vi "Sensors.vi"() -> ()   [LabVIEW 2017]
uses:
  <vilib>/DAQmx/read.llb/DAQmx Read (Analog 1D Wfm NChan 1Samp).vi
  <vilib>/DAQmx/read.llb/DAQmx Read (Analog 1D Wfm NChan NSamp).vi
  <vilib>/DAQmx/miscellaneous.llb/DAQmx Fill In Error Info.vi
panel:
  out "output cluster":T1={"Dynamic Data"=[{"t0"=timestamp(0 s since 1904-01-01), "dt"=1.0, "Y"=[14.93], "attributes"=variant("Alicat_unit"=variant(string "PSIA"), "NI_ChannelName"=variant(string "Absolute Pressure_O2"), "NI_UnitDescription"=variant(string "psi"))}, {"t0"=timestamp(0 s since 1904-01-01), "dt"=1.0, "Y"=[18.45], "attributes"=variant("Alicat_unit"=variant(string "°C"), "NI_ChannelName"=variant(string "Temperature_O2"), "NI_UnitDescription"=variant(string "degC"))}, {"t0"=timestamp(0 s since 1904-01-01), "dt"=1.0, "Y"=[-0.1], "attributes"=variant("Alicat_unit"=variant(string "LPM"), "NI_ChannelName"=variant(string "Volumetric Flow_O2"), "NI_UnitDescription"=variant(string "l/min"))}, {"t0"=timestamp(0 s since 1904-01-01), "dt"=1.0, "Y"=[-0.1], "attributes"=variant("Alicat_unit"=variant(string "SLPM"), "NI_ChannelName"=variant(string "Mass Flow_O2"), "NI_UnitDescription"=variant(string "kg/min"))}, {"t0"=timestamp(0 s since 1904-01-01), "dt"=1.0, "Y"=[104.12], "attributes"=variant("Alicat_unit"=variant(string "PSIA"), "NI_ChannelName"=variant(string "Absolute Pressure_Ar"), "NI_UnitDescription"=variant(string "psi"))}, {"t0"=timestamp(0 s since 1904-01-01), "dt"=1.0, "Y"=[18.33], "attributes"=variant("Alicat_unit"=variant(string "°C"), "NI_ChannelName"=variant(string "Temperature_Ar"), "NI_UnitDescription"=variant(string "degC"))}, {"t0"=timestamp(0 s since 1904-01-01), "dt"=1.0, "Y"=[-0.01], "attributes"=variant("Alicat_unit"=variant(string "LPM"), "NI_ChannelName"=variant(string "Volumetric Flow_Ar"), "NI_UnitDescription"=variant(string "l/min"))}, {"t0"=timestamp(0 s since 1904-01-01), "dt"=1.0, "Y"=[-0.09], "attributes"=variant("Alicat_unit"=variant(string "SLPM"), "NI_ChannelName"=variant(string "Mass Flow_Ar"), "NI_UnitDescription"=variant(string "kg/min"))}, {"t0"=timestamp(3595264812.029535 s since 1904-01-01), "dt"=0.001, "Y"=[14.755946928632032], "attributes"=variant("NI_ChannelName"=variant(string "CCP (Arith. Mean)"), "NI_OriginalChannelName"=variant(string "CCP"), "NI_UnitDescription"=variant(string "psi"))}, {"t0"=timestamp(3595264812.0295486 s since 1904-01-01), "dt"=0.001, "Y"=[-6.516446397140361], "attributes"=variant("NI_ChannelName"=variant(string "PNP (Arith. Mean)"), "NI_OriginalChannelName"=variant(string "PNP"), "NI_UnitDescription"=variant(string "psi"))}, {"t0"=timestamp(3595264812.0295625 s since 1904-01-01), "dt"=0.001, "Y"=[0.00021340766900836388], "attributes"=variant("NI_ChannelName"=variant(string "Fuel Flow (Arith. Mean)"), "NI_OriginalChannelName"=variant(string "Fuel Flow"), "NI_UnitDescription"=variant(string "lpm"))}, {"t0"=timestamp(3595264812.029577 s since 1904-01-01), "dt"=0.001, "Y"=[5.637227790905208], "attributes"=variant("NI_ChannelName"=variant(string "Water Flow (Arith. Mean)"), "NI_OriginalChannelName"=variant(string "Water Flow"), "NI_UnitDescription"=variant(string "lpm"))}, {"t0"=timestamp(3595264811.8456883 s since 1904-01-01), "dt"=0.058823520000000004, "Y"=[17.273451779340505], "attributes"=variant("NI_ChannelName"=variant(string "T_W_in (Arith. Mean)"), "NI_OriginalChannelName"=variant(string "T_W_in"), "NI_UnitDescription"=variant(string "Deg C"))}, {"t0"=timestamp(3595264811.8456883 s since 1904-01-01), "dt"=0.058823520000000004, "Y"=[17.150762268550952], "attributes"=variant("NI_ChannelName"=variant(string "T_W_out (Arith. Mean)"), "NI_OriginalChannelName"=variant(string "T_W_out"), "NI_UnitDescription"=variant(string "Deg C"))}], "Dynamic Data"=[{"t0"=timestamp(3595264811.9295344 s since 1904-01-01), "dt"=0.001, "Y"=[14.699907104909705, 14.618807545369336, 14.756676797002818, 14.19708984696561, 14.124100247221385, 14.926985875335113, 14.813446489437872, 15.218944302517066, 15.332483693323432, 14.23763962484339, 14.480938295748444, 15.308153823748846, 15.05674517518289, 15.227054258957516, 16.946365184439138, 14.205199802527325, 15.105404913088343, 16.02993998150081, 15.65688196038274, 14.975645612567924, 16.005610110100243, 15.997500152980955, 14.456608428376889, 15.583892349309288, 15.600112262831665, 14.878326138354218, 14.278189402894249, 15.283823954237583, 14.967535656344957, 14.618807545369336, 15.024305350052806, 14.570147809979424, 15.664991917204041, 14.991865525034875, 14.52959803067921, 15.235164215405, 14.975645612567924, 13.92946131730504, 13.18334545594982, 14.78100666514738, 14.010560870953888, 14.043000692606519, 14.772896709092215, 14.667467281009941, 12.721078049068659, 14.578257765860343, 14.651247369101874, 12.429119698153222, 14.983755568797896, 13.961901138681867, 12.891387091145475, 14.967535656344957, 14.626917501292006, 13.483413784528253, 14.245749580439714, 14.464718384160463, 13.92946131730504, 14.894546050653211, 15.05674517518289, 14.059220603474259, 14.821556445527968, 14.85399626995818, 14.886436094500219, 14.894546050653211, 15.218944302517066, 13.759152256884029, 14.91887591915414, 15.48657286876847, 15.081075044104047, 15.251384128321057, 15.373033476088615, 15.202724389657241, 14.94320578771805, 15.778531313445832, 14.85399626995818, 15.081075044104047, 15.291933910734308, 15.397363345832254, 15.227054258957516, 15.608222219603455, 15.097294956753224, 14.261969491653119, 14.578257765860343, 14.39172878235832, 14.85399626995818, 14.31873918111829, 15.794751227308033, 14.302519269807874, 12.680528277585267, 14.537707986525348, 14.78100666514738, 14.991865525034875, 14.821556445527968, 14.334959092456415, 14.213309758095953, 14.643137413158279, 15.129734782135792, 13.742932346525912, 14.6106975894536, 15.664991917204041], "attributes"=variant("NI_ChannelName"=variant(string "CCP"), "NI_UnitDescription"=variant(string "psi"))}, {"t0"=timestamp(3595264811.9295487 s since 1904-01-01), "dt"=0.001, "Y"=[-6.5968159210350805, -5.331665115123144, -6.767124674607722, -7.286160863340072, -7.067192473529879, -6.848224080348615, -6.6698053871039065, -6.118329411843284, -6.523826454587585, -6.7752346152027485, -5.988570355674682, -6.864443961440983, -6.823894258675196, -6.710355090312085, -7.099632235195543, -7.213171400443514, -7.278050923036652, -6.653585505787973, -7.002312949976542, -7.424029847795147, -6.66169544644827, -6.66169544644827, -6.215648703175461, -6.823894258675196, -6.24808846680186, -6.548156276778862, -6.540046336053116, -6.2318685849980895, -6.6698053871039065, -6.637365624453359, -6.710355090312085, -6.069669765922043, -6.126439352813605, -7.448359668443629, -5.323555173685449, -6.686025268401167, -5.347884997984096, -6.888773783044712, -5.469534118828456, -6.361627638900849, -6.304858052966658, -6.66169544644827, -6.7752346152027485, -7.310490684222756, -7.407809967339887, -6.832004199237652, -6.483276750841782, -6.929323485624721, -7.156401817932583, -5.769601945636374, -7.099632235195543, -5.88314112164425, -6.986093069041907, -6.9049936640906395, -7.042862652232081, -6.345407757228877, -6.280528230352857, -6.23997852590233, -6.637365624453359, -7.675437992510332, -6.085889647914705, -6.38595746137355, -6.085889647914705, -5.850701357165718, -6.880663842514778, -5.793931769145161, -6.613035802416412, -5.485754001526104, -5.802041710305232, -5.907470944953253, -6.767124674607722, -5.5181937668638525, -6.613035802416412, -6.2643083485867805, -6.929323485624721, -7.261831042415984, -6.564376158216312, -8.218803967769759, -5.88314112164425, -6.28863817122884, -6.848224080348615, -6.986093069041907, -6.937433426126795, -7.123962056396266, -6.442727046978796, -5.915580886046762, -6.045339942897556, -6.645475565122993, -6.069669765922043, -6.085889647914705, -6.05344988391046, -6.832004199237652, -5.948020650373287, -5.996680296720733, -6.004790237762052, -6.686025268401167, -5.2992253493435015, -7.018532830892646, -5.396544646451538, -6.6698053871039065], "attributes"=variant("NI_ChannelName"=variant(string "PNP"), "NI_UnitDescription"=variant(string "psi"))}, {"t0"=timestamp(3595264811.9295626 s since 1904-01-01), "dt"=0.001, "Y"=[0.0012713094454450263, -0.00038920178427442886, 0.00019268675156380866, 0.0003629955943209723, 0.00012172473414999441, 0.0014274258925409539, 0.00030622597991726563, 9.333992725056584e-05, 3.6570313564923684e-05, 0.00034880319070584864, 0.0002068791550749044, -3.439170332994457e-05, 0.00019268675156380866, -0.0008007814708233113, 0.00019268675156380866, 0.00013591713761386404, -0.00023308534938290548, -0.0007440118593533968, 0.00027784117277217246, 5.076271697218582e-05, -4.858410668064084e-05, -4.858410668064084e-05, 0.00015010954108719832, -0.0010562447205899328, -0.00017631573641313514, 0.000263648769213809, 9.333992725056584e-05, 0.0017538511947627622, 9.333992725056584e-05, 5.076271697218582e-05, 9.333992725056584e-05, 0.0003913804015796135, 7.914752381500689e-05, 0.0012996942539217904, 0.00010753233069556167, 9.333992725056584e-05, 0.00037718799794556057, 0.0010868081912780159, 0.00015010954108719832, -6.006896600282974e-06, -0.00047435620282741675, 7.914752381500689e-05, 0.00015010954108719832, 3.6570313564923684e-05, 0.00027784117277217246, 0.0012996942539217904, 0.00016430194456995562, 0.00033461078710018965, 0.0002352639621254482, 5.076271697218582e-05, 2.2377910167098447e-05, -2.019929996982528e-05, 5.076271697218582e-05, 0.0002068791550749044, -6.277651002191409e-05, 0.0009732689587464011, -6.006896600282974e-06, 6.495512038888485e-05, 6.495512038888485e-05, 7.914752381500689e-05, 0.00033461078710018965, -7.696891335376432e-05, 6.495512038888485e-05, 0.002449279029525811, 0.0007887677071832383, 0.0002210715585954509, -4.858410668064084e-05, 0.0002068791550749044, -2.019929996982528e-05, 0.00034880319070584864, 0.00013591713761386404, -7.696891335376432e-05, -0.0022625989149816506, -0.00016212333314716276, 0.0003629955943209723, 0.0001784943480621637, -0.00023308534938290548, 0.0001784943480621637, 6.495512038888485e-05, 0.00047653482358286925, 2.2377910167098447e-05, -3.439170332994457e-05, 0.002349932194567847, 0.00193835245478928, 0.0006184588610133601, 0.00024945636566489626, 0.00024945636566489626, -0.0001053537199892235, 0.00033461078710018965, 0.00019268675156380866, 0.0001784943480621637, 8.185506778696228e-06, 0.0006610360724275677, 0.0005474968421795429, -7.696891335376432e-05, -3.439170332994457e-05, 0.00019268675156380866, 0.0001784943480621637, -0.00016212333314716276, -0.00019050813966967062], "attributes"=variant("NI_ChannelName"=variant(string "Fuel Flow"), "NI_UnitDescription"=variant(string "lpm"))}, {"t0"=timestamp(3595264811.929577 s since 1904-01-01), "dt"=0.001, "Y"=[5.572084656080217, 5.681568898491807, 5.160423935874966, 5.714414171906223, 5.604929928432683, 5.591791819453621, 5.661861734596575, 5.883019913826618, 5.642154570816197, 5.61368866778029, 5.664051419468147, 5.427565461482891, 5.688137953149105, 5.740690390868342, 5.668430789215548, 5.12757866774301, 5.714414171906223, 5.604929928432683, 5.720983226627516, 5.326839965809641, 5.707845117197739, 5.5961711891076655, 5.644344255675015, 5.539239384044607, 5.6859482682619165, 6.421682471798005, 5.753828500426406, 5.580843395343192, 5.666241104341139, 6.318767260726264, 5.440703569830947, 5.554567177621844, 5.5611362320331805, 5.587412449805222, 5.212976365524704, 5.7472594456409505, 5.648723625396905, 5.635585516248232, 6.101988422603111, 5.5523774928208764, 5.618068037462568, 6.441389640252797, 5.679379213608882, 5.740690390868342, 5.587412449805222, 5.701276062502065, 5.661861734596575, 5.624637091996585, 5.703465747399199, 5.241442265247469, 5.681568898491807, 5.699086377606348, 5.519532220974999, 5.784484089595206, 5.692517322927739, 5.661861734596575, 5.7056554322977595, 5.348736812445613, 4.317395482050515, 5.451651993492663, 5.495445688488638, 5.727552281361631, 5.637775201102804, 5.644344255675015, 5.674999843847291, 5.690327638037711, 5.484497264687218, 6.432630898702322, 5.1560445667729935, 5.5523774928208764, 5.591791819453621, 5.683758583376151, 5.6859482682619165, 5.679379213608882, 5.674999843847291, 5.913675504181955, 5.191079519741636, 5.753828500426406, 5.742880075791118, 5.578653710525335, 5.712224487001971, 5.661861734596575, 5.631206146543328, 5.688137953149105, 5.593981504279939, 5.670620474091376, 5.629016461692999, 5.212976365524704, 6.412923730301547, 5.712224487001971, 5.639964885958791, 5.6509133102599725, 5.688137953149105, 5.653102995124461, 5.574274340893848, 5.079405608369558, 5.896158023944262, 5.655292679990361, 5.670620474091376, 5.668430789215548], "attributes"=variant("NI_ChannelName"=variant(string "Water Flow"), "NI_UnitDescription"=variant(string "lpm"))}, {"t0"=timestamp(3595264811.728041 s since 1904-01-01), "dt"=0.058823520000000004, "Y"=[17.273340401742463, 17.273563156938543], "attributes"=variant("NI_ChannelName"=variant(string "T_W_in"), "NI_UnitDescription"=variant(string "Deg C"))}, {"t0"=timestamp(3595264811.728041 s since 1904-01-01), "dt"=0.058823520000000004, "Y"=[17.14969975423883, 17.151824782863073], "attributes"=variant("NI_ChannelName"=variant(string "T_W_out"), "NI_UnitDescription"=variant(string "Deg C"))}], "Dynamic Data"=[{"t0"=timestamp(3595264811.860325 s since 1904-01-01), "dt"=0.058823520000000004, "Y"=[16.92806090865619], "attributes"=variant("NI_ChannelName"=variant(string "T_Sample (Arith. Mean)"), "NI_OriginalChannelName"=variant(string "T_Sample"), "NI_UnitDescription"=variant(string "Deg C"))}], "Dynamic Data Type"=[{"t0"=timestamp(3595264811.7426777 s since 1904-01-01), "dt"=0.058823520000000004, "Y"=[16.929019700348153, 16.927102116964225], "attributes"=variant("NI_ChannelName"=variant(string "T_Sample"), "NI_UnitDescription"=variant(string "Deg C"))}]}
  out "Non HVOF process Raw":dynamicdata(graph)=[{"t0"=timestamp(3595264811.7426777 s since 1904-01-01), "dt"=0.058823520000000004, "Y"=[16.929019700348153, 16.927102116964225], "attributes"=variant("NI_ChannelName"=variant(string "T_Sample"), "NI_UnitDescription"=variant(string "Deg C"))}]
  out "HVOF Process Raw":dynamicdata(graph)=[{"t0"=timestamp(3595264811.9295344 s since 1904-01-01), "dt"=0.001, "Y"=[14.699907104909705, 14.618807545369336, 14.756676797002818, 14.19708984696561, 14.124100247221385, 14.926985875335113, 14.813446489437872, 15.218944302517066, 15.332483693323432, 14.23763962484339, 14.480938295748444, 15.308153823748846, 15.05674517518289, 15.227054258957516, 16.946365184439138, 14.205199802527325, 15.105404913088343, 16.02993998150081, 15.65688196038274, 14.975645612567924, 16.005610110100243, 15.997500152980955, 14.456608428376889, 15.583892349309288, 15.600112262831665, 14.878326138354218, 14.278189402894249, 15.283823954237583, 14.967535656344957, 14.618807545369336, 15.024305350052806, 14.570147809979424, 15.664991917204041, 14.991865525034875, 14.52959803067921, 15.235164215405, 14.975645612567924, 13.92946131730504, 13.18334545594982, 14.78100666514738, 14.010560870953888, 14.043000692606519, 14.772896709092215, 14.667467281009941, 12.721078049068659, 14.578257765860343, 14.651247369101874, 12.429119698153222, 14.983755568797896, 13.961901138681867, 12.891387091145475, 14.967535656344957, 14.626917501292006, 13.483413784528253, 14.245749580439714, 14.464718384160463, 13.92946131730504, 14.894546050653211, 15.05674517518289, 14.059220603474259, 14.821556445527968, 14.85399626995818, 14.886436094500219, 14.894546050653211, 15.218944302517066, 13.759152256884029, 14.91887591915414, 15.48657286876847, 15.081075044104047, 15.251384128321057, 15.373033476088615, 15.202724389657241, 14.94320578771805, 15.778531313445832, 14.85399626995818, 15.081075044104047, 15.291933910734308, 15.397363345832254, 15.227054258957516, 15.608222219603455, 15.097294956753224, 14.261969491653119, 14.578257765860343, 14.39172878235832, 14.85399626995818, 14.31873918111829, 15.794751227308033, 14.302519269807874, 12.680528277585267, 14.537707986525348, 14.78100666514738, 14.991865525034875, 14.821556445527968, 14.334959092456415, 14.213309758095953, 14.643137413158279, 15.129734782135792, 13.742932346525912, 14.6106975894536, 15.664991917204041], "attributes"=variant("NI_ChannelName"=variant(string "CCP"), "NI_UnitDescription"=variant(string "psi"))}, {"t0"=timestamp(3595264811.9295487 s since 1904-01-01), "dt"=0.001, "Y"=[-6.5968159210350805, -5.331665115123144, -6.767124674607722, -7.286160863340072, -7.067192473529879, -6.848224080348615, -6.6698053871039065, -6.118329411843284, -6.523826454587585, -6.7752346152027485, -5.988570355674682, -6.864443961440983, -6.823894258675196, -6.710355090312085, -7.099632235195543, -7.213171400443514, -7.278050923036652, -6.653585505787973, -7.002312949976542, -7.424029847795147, -6.66169544644827, -6.66169544644827, -6.215648703175461, -6.823894258675196, -6.24808846680186, -6.548156276778862, -6.540046336053116, -6.2318685849980895, -6.6698053871039065, -6.637365624453359, -6.710355090312085, -6.069669765922043, -6.126439352813605, -7.448359668443629, -5.323555173685449, -6.686025268401167, -5.347884997984096, -6.888773783044712, -5.469534118828456, -6.361627638900849, -6.304858052966658, -6.66169544644827, -6.7752346152027485, -7.310490684222756, -7.407809967339887, -6.832004199237652, -6.483276750841782, -6.929323485624721, -7.156401817932583, -5.769601945636374, -7.099632235195543, -5.88314112164425, -6.986093069041907, -6.9049936640906395, -7.042862652232081, -6.345407757228877, -6.280528230352857, -6.23997852590233, -6.637365624453359, -7.675437992510332, -6.085889647914705, -6.38595746137355, -6.085889647914705, -5.850701357165718, -6.880663842514778, -5.793931769145161, -6.613035802416412, -5.485754001526104, -5.802041710305232, -5.907470944953253, -6.767124674607722, -5.5181937668638525, -6.613035802416412, -6.2643083485867805, -6.929323485624721, -7.261831042415984, -6.564376158216312, -8.218803967769759, -5.88314112164425, -6.28863817122884, -6.848224080348615, -6.986093069041907, -6.937433426126795, -7.123962056396266, -6.442727046978796, -5.915580886046762, -6.045339942897556, -6.645475565122993, -6.069669765922043, -6.085889647914705, -6.05344988391046, -6.832004199237652, -5.948020650373287, -5.996680296720733, -6.004790237762052, -6.686025268401167, -5.2992253493435015, -7.018532830892646, -5.396544646451538, -6.6698053871039065], "attributes"=variant("NI_ChannelName"=variant(string "PNP"), "NI_UnitDescription"=variant(string "psi"))}, {"t0"=timestamp(3595264811.9295626 s since 1904-01-01), "dt"=0.001, "Y"=[0.0012713094454450263, -0.00038920178427442886, 0.00019268675156380866, 0.0003629955943209723, 0.00012172473414999441, 0.0014274258925409539, 0.00030622597991726563, 9.333992725056584e-05, 3.6570313564923684e-05, 0.00034880319070584864, 0.0002068791550749044, -3.439170332994457e-05, 0.00019268675156380866, -0.0008007814708233113, 0.00019268675156380866, 0.00013591713761386404, -0.00023308534938290548, -0.0007440118593533968, 0.00027784117277217246, 5.076271697218582e-05, -4.858410668064084e-05, -4.858410668064084e-05, 0.00015010954108719832, -0.0010562447205899328, -0.00017631573641313514, 0.000263648769213809, 9.333992725056584e-05, 0.0017538511947627622, 9.333992725056584e-05, 5.076271697218582e-05, 9.333992725056584e-05, 0.0003913804015796135, 7.914752381500689e-05, 0.0012996942539217904, 0.00010753233069556167, 9.333992725056584e-05, 0.00037718799794556057, 0.0010868081912780159, 0.00015010954108719832, -6.006896600282974e-06, -0.00047435620282741675, 7.914752381500689e-05, 0.00015010954108719832, 3.6570313564923684e-05, 0.00027784117277217246, 0.0012996942539217904, 0.00016430194456995562, 0.00033461078710018965, 0.0002352639621254482, 5.076271697218582e-05, 2.2377910167098447e-05, -2.019929996982528e-05, 5.076271697218582e-05, 0.0002068791550749044, -6.277651002191409e-05, 0.0009732689587464011, -6.006896600282974e-06, 6.495512038888485e-05, 6.495512038888485e-05, 7.914752381500689e-05, 0.00033461078710018965, -7.696891335376432e-05, 6.495512038888485e-05, 0.002449279029525811, 0.0007887677071832383, 0.0002210715585954509, -4.858410668064084e-05, 0.0002068791550749044, -2.019929996982528e-05, 0.00034880319070584864, 0.00013591713761386404, -7.696891335376432e-05, -0.0022625989149816506, -0.00016212333314716276, 0.0003629955943209723, 0.0001784943480621637, -0.00023308534938290548, 0.0001784943480621637, 6.495512038888485e-05, 0.00047653482358286925, 2.2377910167098447e-05, -3.439170332994457e-05, 0.002349932194567847, 0.00193835245478928, 0.0006184588610133601, 0.00024945636566489626, 0.00024945636566489626, -0.0001053537199892235, 0.00033461078710018965, 0.00019268675156380866, 0.0001784943480621637, 8.185506778696228e-06, 0.0006610360724275677, 0.0005474968421795429, -7.696891335376432e-05, -3.439170332994457e-05, 0.00019268675156380866, 0.0001784943480621637, -0.00016212333314716276, -0.00019050813966967062], "attributes"=variant("NI_ChannelName"=variant(string "Fuel Flow"), "NI_UnitDescription"=variant(string "lpm"))}, {"t0"=timestamp(3595264811.929577 s since 1904-01-01), "dt"=0.001, "Y"=[5.572084656080217, 5.681568898491807, 5.160423935874966, 5.714414171906223, 5.604929928432683, 5.591791819453621, 5.661861734596575, 5.883019913826618, 5.642154570816197, 5.61368866778029, 5.664051419468147, 5.427565461482891, 5.688137953149105, 5.740690390868342, 5.668430789215548, 5.12757866774301, 5.714414171906223, 5.604929928432683, 5.720983226627516, 5.326839965809641, 5.707845117197739, 5.5961711891076655, 5.644344255675015, 5.539239384044607, 5.6859482682619165, 6.421682471798005, 5.753828500426406, 5.580843395343192, 5.666241104341139, 6.318767260726264, 5.440703569830947, 5.554567177621844, 5.5611362320331805, 5.587412449805222, 5.212976365524704, 5.7472594456409505, 5.648723625396905, 5.635585516248232, 6.101988422603111, 5.5523774928208764, 5.618068037462568, 6.441389640252797, 5.679379213608882, 5.740690390868342, 5.587412449805222, 5.701276062502065, 5.661861734596575, 5.624637091996585, 5.703465747399199, 5.241442265247469, 5.681568898491807, 5.699086377606348, 5.519532220974999, 5.784484089595206, 5.692517322927739, 5.661861734596575, 5.7056554322977595, 5.348736812445613, 4.317395482050515, 5.451651993492663, 5.495445688488638, 5.727552281361631, 5.637775201102804, 5.644344255675015, 5.674999843847291, 5.690327638037711, 5.484497264687218, 6.432630898702322, 5.1560445667729935, 5.5523774928208764, 5.591791819453621, 5.683758583376151, 5.6859482682619165, 5.679379213608882, 5.674999843847291, 5.913675504181955, 5.191079519741636, 5.753828500426406, 5.742880075791118, 5.578653710525335, 5.712224487001971, 5.661861734596575, 5.631206146543328, 5.688137953149105, 5.593981504279939, 5.670620474091376, 5.629016461692999, 5.212976365524704, 6.412923730301547, 5.712224487001971, 5.639964885958791, 5.6509133102599725, 5.688137953149105, 5.653102995124461, 5.574274340893848, 5.079405608369558, 5.896158023944262, 5.655292679990361, 5.670620474091376, 5.668430789215548], "attributes"=variant("NI_ChannelName"=variant(string "Water Flow"), "NI_UnitDescription"=variant(string "lpm"))}, {"t0"=timestamp(3595264811.728041 s since 1904-01-01), "dt"=0.058823520000000004, "Y"=[17.273340401742463, 17.273563156938543], "attributes"=variant("NI_ChannelName"=variant(string "T_W_in"), "NI_UnitDescription"=variant(string "Deg C"))}, {"t0"=timestamp(3595264811.728041 s since 1904-01-01), "dt"=0.058823520000000004, "Y"=[17.14969975423883, 17.151824782863073], "attributes"=variant("NI_ChannelName"=variant(string "T_W_out"), "NI_UnitDescription"=variant(string "Deg C"))}]
  out "Non HVOF process":dynamicdata(graph)=[{"t0"=timestamp(3595264811.860325 s since 1904-01-01), "dt"=0.058823520000000004, "Y"=[16.92806090865619], "attributes"=variant("NI_ChannelName"=variant(string "T_Sample (Arith. Mean)"), "NI_OriginalChannelName"=variant(string "T_Sample"), "NI_UnitDescription"=variant(string "Deg C"))}]
  out "Raw Data DAQ 1":waveform(dbl)[](graph)=[{"t0"=timestamp(3595264811.9295344 s since 1904-01-01), "dt"=0.001, "Y"=[14.699907104909705, 14.618807545369336, 14.756676797002818, 14.19708984696561, 14.124100247221385, 14.926985875335113, 14.813446489437872, 15.218944302517066, 15.332483693323432, 14.23763962484339, 14.480938295748444, 15.308153823748846, 15.05674517518289, 15.227054258957516, 16.946365184439138, 14.205199802527325, 15.105404913088343, 16.02993998150081, 15.65688196038274, 14.975645612567924, 16.005610110100243, 15.997500152980955, 14.456608428376889, 15.583892349309288, 15.600112262831665, 14.878326138354218, 14.278189402894249, 15.283823954237583, 14.967535656344957, 14.618807545369336, 15.024305350052806, 14.570147809979424, 15.664991917204041, 14.991865525034875, 14.52959803067921, 15.235164215405, 14.975645612567924, 13.92946131730504, 13.18334545594982, 14.78100666514738, 14.010560870953888, 14.043000692606519, 14.772896709092215, 14.667467281009941, 12.721078049068659, 14.578257765860343, 14.651247369101874, 12.429119698153222, 14.983755568797896, 13.961901138681867, 12.891387091145475, 14.967535656344957, 14.626917501292006, 13.483413784528253, 14.245749580439714, 14.464718384160463, 13.92946131730504, 14.894546050653211, 15.05674517518289, 14.059220603474259, 14.821556445527968, 14.85399626995818, 14.886436094500219, 14.894546050653211, 15.218944302517066, 13.759152256884029, 14.91887591915414, 15.48657286876847, 15.081075044104047, 15.251384128321057, 15.373033476088615, 15.202724389657241, 14.94320578771805, 15.778531313445832, 14.85399626995818, 15.081075044104047, 15.291933910734308, 15.397363345832254, 15.227054258957516, 15.608222219603455, 15.097294956753224, 14.261969491653119, 14.578257765860343, 14.39172878235832, 14.85399626995818, 14.31873918111829, 15.794751227308033, 14.302519269807874, 12.680528277585267, 14.537707986525348, 14.78100666514738, 14.991865525034875, 14.821556445527968, 14.334959092456415, 14.213309758095953, 14.643137413158279, 15.129734782135792, 13.742932346525912, 14.6106975894536, 15.664991917204041], "attributes"=variant("NI_ChannelName"=variant(string "CCP"), "NI_UnitDescription"=variant(string "psi"))}, {"t0"=timestamp(3595264811.9295487 s since 1904-01-01), "dt"=0.001, "Y"=[-6.5968159210350805, -5.331665115123144, -6.767124674607722, -7.286160863340072, -7.067192473529879, -6.848224080348615, -6.6698053871039065, -6.118329411843284, -6.523826454587585, -6.7752346152027485, -5.988570355674682, -6.864443961440983, -6.823894258675196, -6.710355090312085, -7.099632235195543, -7.213171400443514, -7.278050923036652, -6.653585505787973, -7.002312949976542, -7.424029847795147, -6.66169544644827, -6.66169544644827, -6.215648703175461, -6.823894258675196, -6.24808846680186, -6.548156276778862, -6.540046336053116, -6.2318685849980895, -6.6698053871039065, -6.637365624453359, -6.710355090312085, -6.069669765922043, -6.126439352813605, -7.448359668443629, -5.323555173685449, -6.686025268401167, -5.347884997984096, -6.888773783044712, -5.469534118828456, -6.361627638900849, -6.304858052966658, -6.66169544644827, -6.7752346152027485, -7.310490684222756, -7.407809967339887, -6.832004199237652, -6.483276750841782, -6.929323485624721, -7.156401817932583, -5.769601945636374, -7.099632235195543, -5.88314112164425, -6.986093069041907, -6.9049936640906395, -7.042862652232081, -6.345407757228877, -6.280528230352857, -6.23997852590233, -6.637365624453359, -7.675437992510332, -6.085889647914705, -6.38595746137355, -6.085889647914705, -5.850701357165718, -6.880663842514778, -5.793931769145161, -6.613035802416412, -5.485754001526104, -5.802041710305232, -5.907470944953253, -6.767124674607722, -5.5181937668638525, -6.613035802416412, -6.2643083485867805, -6.929323485624721, -7.261831042415984, -6.564376158216312, -8.218803967769759, -5.88314112164425, -6.28863817122884, -6.848224080348615, -6.986093069041907, -6.937433426126795, -7.123962056396266, -6.442727046978796, -5.915580886046762, -6.045339942897556, -6.645475565122993, -6.069669765922043, -6.085889647914705, -6.05344988391046, -6.832004199237652, -5.948020650373287, -5.996680296720733, -6.004790237762052, -6.686025268401167, -5.2992253493435015, -7.018532830892646, -5.396544646451538, -6.6698053871039065], "attributes"=variant("NI_ChannelName"=variant(string "PNP"), "NI_UnitDescription"=variant(string "psi"))}, {"t0"=timestamp(3595264811.9295626 s since 1904-01-01), "dt"=0.001, "Y"=[0.0012713094454450263, -0.00038920178427442886, 0.00019268675156380866, 0.0003629955943209723, 0.00012172473414999441, 0.0014274258925409539, 0.00030622597991726563, 9.333992725056584e-05, 3.6570313564923684e-05, 0.00034880319070584864, 0.0002068791550749044, -3.439170332994457e-05, 0.00019268675156380866, -0.0008007814708233113, 0.00019268675156380866, 0.00013591713761386404, -0.00023308534938290548, -0.0007440118593533968, 0.00027784117277217246, 5.076271697218582e-05, -4.858410668064084e-05, -4.858410668064084e-05, 0.00015010954108719832, -0.0010562447205899328, -0.00017631573641313514, 0.000263648769213809, 9.333992725056584e-05, 0.0017538511947627622, 9.333992725056584e-05, 5.076271697218582e-05, 9.333992725056584e-05, 0.0003913804015796135, 7.914752381500689e-05, 0.0012996942539217904, 0.00010753233069556167, 9.333992725056584e-05, 0.00037718799794556057, 0.0010868081912780159, 0.00015010954108719832, -6.006896600282974e-06, -0.00047435620282741675, 7.914752381500689e-05, 0.00015010954108719832, 3.6570313564923684e-05, 0.00027784117277217246, 0.0012996942539217904, 0.00016430194456995562, 0.00033461078710018965, 0.0002352639621254482, 5.076271697218582e-05, 2.2377910167098447e-05, -2.019929996982528e-05, 5.076271697218582e-05, 0.0002068791550749044, -6.277651002191409e-05, 0.0009732689587464011, -6.006896600282974e-06, 6.495512038888485e-05, 6.495512038888485e-05, 7.914752381500689e-05, 0.00033461078710018965, -7.696891335376432e-05, 6.495512038888485e-05, 0.002449279029525811, 0.0007887677071832383, 0.0002210715585954509, -4.858410668064084e-05, 0.0002068791550749044, -2.019929996982528e-05, 0.00034880319070584864, 0.00013591713761386404, -7.696891335376432e-05, -0.0022625989149816506, -0.00016212333314716276, 0.0003629955943209723, 0.0001784943480621637, -0.00023308534938290548, 0.0001784943480621637, 6.495512038888485e-05, 0.00047653482358286925, 2.2377910167098447e-05, -3.439170332994457e-05, 0.002349932194567847, 0.00193835245478928, 0.0006184588610133601, 0.00024945636566489626, 0.00024945636566489626, -0.0001053537199892235, 0.00033461078710018965, 0.00019268675156380866, 0.0001784943480621637, 8.185506778696228e-06, 0.0006610360724275677, 0.0005474968421795429, -7.696891335376432e-05, -3.439170332994457e-05, 0.00019268675156380866, 0.0001784943480621637, -0.00016212333314716276, -0.00019050813966967062], "attributes"=variant("NI_ChannelName"=variant(string "Fuel Flow"), "NI_UnitDescription"=variant(string "lpm"))}, {"t0"=timestamp(3595264811.929577 s since 1904-01-01), "dt"=0.001, "Y"=[5.572084656080217, 5.681568898491807, 5.160423935874966, 5.714414171906223, 5.604929928432683, 5.591791819453621, 5.661861734596575, 5.883019913826618, 5.642154570816197, 5.61368866778029, 5.664051419468147, 5.427565461482891, 5.688137953149105, 5.740690390868342, 5.668430789215548, 5.12757866774301, 5.714414171906223, 5.604929928432683, 5.720983226627516, 5.326839965809641, 5.707845117197739, 5.5961711891076655, 5.644344255675015, 5.539239384044607, 5.6859482682619165, 6.421682471798005, 5.753828500426406, 5.580843395343192, 5.666241104341139, 6.318767260726264, 5.440703569830947, 5.554567177621844, 5.5611362320331805, 5.587412449805222, 5.212976365524704, 5.7472594456409505, 5.648723625396905, 5.635585516248232, 6.101988422603111, 5.5523774928208764, 5.618068037462568, 6.441389640252797, 5.679379213608882, 5.740690390868342, 5.587412449805222, 5.701276062502065, 5.661861734596575, 5.624637091996585, 5.703465747399199, 5.241442265247469, 5.681568898491807, 5.699086377606348, 5.519532220974999, 5.784484089595206, 5.692517322927739, 5.661861734596575, 5.7056554322977595, 5.348736812445613, 4.317395482050515, 5.451651993492663, 5.495445688488638, 5.727552281361631, 5.637775201102804, 5.644344255675015, 5.674999843847291, 5.690327638037711, 5.484497264687218, 6.432630898702322, 5.1560445667729935, 5.5523774928208764, 5.591791819453621, 5.683758583376151, 5.6859482682619165, 5.679379213608882, 5.674999843847291, 5.913675504181955, 5.191079519741636, 5.753828500426406, 5.742880075791118, 5.578653710525335, 5.712224487001971, 5.661861734596575, 5.631206146543328, 5.688137953149105, 5.593981504279939, 5.670620474091376, 5.629016461692999, 5.212976365524704, 6.412923730301547, 5.712224487001971, 5.639964885958791, 5.6509133102599725, 5.688137953149105, 5.653102995124461, 5.574274340893848, 5.079405608369558, 5.896158023944262, 5.655292679990361, 5.670620474091376, 5.668430789215548], "attributes"=variant("NI_ChannelName"=variant(string "Water Flow"), "NI_UnitDescription"=variant(string "lpm"))}] caption="data"
  out "file size TDMS":dbl=122.615234375
  in  "Save Data TDMS":bool=TRUE
  in  "Stop":bool
  out "HVOF Process":dynamicdata(graph)=[{"t0"=timestamp(0 s since 1904-01-01), "dt"=1.0, "Y"=[14.93], "attributes"=variant("Alicat_unit"=variant(string "PSIA"), "NI_ChannelName"=variant(string "Absolute Pressure_O2"), "NI_UnitDescription"=variant(string "psi"))}, {"t0"=timestamp(0 s since 1904-01-01), "dt"=1.0, "Y"=[18.45], "attributes"=variant("Alicat_unit"=variant(string "°C"), "NI_ChannelName"=variant(string "Temperature_O2"), "NI_UnitDescription"=variant(string "degC"))}, {"t0"=timestamp(0 s since 1904-01-01), "dt"=1.0, "Y"=[-0.1], "attributes"=variant("Alicat_unit"=variant(string "LPM"), "NI_ChannelName"=variant(string "Volumetric Flow_O2"), "NI_UnitDescription"=variant(string "l/min"))}, {"t0"=timestamp(0 s since 1904-01-01), "dt"=1.0, "Y"=[-0.1], "attributes"=variant("Alicat_unit"=variant(string "SLPM"), "NI_ChannelName"=variant(string "Mass Flow_O2"), "NI_UnitDescription"=variant(string "kg/min"))}, {"t0"=timestamp(0 s since 1904-01-01), "dt"=1.0, "Y"=[104.12], "attributes"=variant("Alicat_unit"=variant(string "PSIA"), "NI_ChannelName"=variant(string "Absolute Pressure_Ar"), "NI_UnitDescription"=variant(string "psi"))}, {"t0"=timestamp(0 s since 1904-01-01), "dt"=1.0, "Y"=[18.33], "attributes"=variant("Alicat_unit"=variant(string "°C"), "NI_ChannelName"=variant(string "Temperature_Ar"), "NI_UnitDescription"=variant(string "degC"))}, {"t0"=timestamp(0 s since 1904-01-01), "dt"=1.0, "Y"=[-0.01], "attributes"=variant("Alicat_unit"=variant(string "LPM"), "NI_ChannelName"=variant(string "Volumetric Flow_Ar"), "NI_UnitDescription"=variant(string "l/min"))}, {"t0"=timestamp(0 s since 1904-01-01), "dt"=1.0, "Y"=[-0.09], "attributes"=variant("Alicat_unit"=variant(string "SLPM"), "NI_ChannelName"=variant(string "Mass Flow_Ar"), "NI_UnitDescription"=variant(string "kg/min"))}, {"t0"=timestamp(3595264812.029535 s since 1904-01-01), "dt"=0.001, "Y"=[14.755946928632032], "attributes"=variant("NI_ChannelName"=variant(string "CCP (Arith. Mean)"), "NI_OriginalChannelName"=variant(string "CCP"), "NI_UnitDescription"=variant(string "psi"))}, {"t0"=timestamp(3595264812.0295486 s since 1904-01-01), "dt"=0.001, "Y"=[-6.516446397140361], "attributes"=variant("NI_ChannelName"=variant(string "PNP (Arith. Mean)"), "NI_OriginalChannelName"=variant(string "PNP"), "NI_UnitDescription"=variant(string "psi"))}, {"t0"=timestamp(3595264812.0295625 s since 1904-01-01), "dt"=0.001, "Y"=[0.00021340766900836388], "attributes"=variant("NI_ChannelName"=variant(string "Fuel Flow (Arith. Mean)"), "NI_OriginalChannelName"=variant(string "Fuel Flow"), "NI_UnitDescription"=variant(string "lpm"))}, {"t0"=timestamp(3595264812.029577 s since 1904-01-01), "dt"=0.001, "Y"=[5.637227790905208], "attributes"=variant("NI_ChannelName"=variant(string "Water Flow (Arith. Mean)"), "NI_OriginalChannelName"=variant(string "Water Flow"), "NI_UnitDescription"=variant(string "lpm"))}, {"t0"=timestamp(3595264811.8456883 s since 1904-01-01), "dt"=0.058823520000000004, "Y"=[17.273451779340505], "attributes"=variant("NI_ChannelName"=variant(string "T_W_in (Arith. Mean)"), "NI_OriginalChannelName"=variant(string "T_W_in"), "NI_UnitDescription"=variant(string "Deg C"))}, {"t0"=timestamp(3595264811.8456883 s since 1904-01-01), "dt"=0.058823520000000004, "Y"=[17.150762268550952], "attributes"=variant("NI_ChannelName"=variant(string "T_W_out (Arith. Mean)"), "NI_OriginalChannelName"=variant(string "T_W_out"), "NI_UnitDescription"=variant(string "Deg C"))}]
  in  "Tab Control":enum32{"File", "Extra"}(tab)=enum."Extra"
  in  "Filename":string="Run1_Sensors"
  out "file path":path=path "C:/Users/aspitarl/Google Drive/NETL/Labview/Learn/TDMS test/2017-12-04/Run1_Sensors.tdms"
  in  "base path":path=path "C:/Users/aspitarl/Google Drive/NETL/Labview/Learn/TDMS test"
  out "Elapsed Time [ms]":dbl=104.01010513305664 caption="Elapsed Time (s)"
  out "Measurements\nper second":dbl=9.614450429799428
  in  "Minimum time between \nreadings [ms]":u32
  in  "O2 [ A-19200-COM7]":T2={" ID"="A", "Baud"=enum."19200", "VISA Sesssion In"="COM4"}
  in  "AR [ B-19200-COM8]":T3={" ID"="B", "Baud "=enum."19200", "VISA Sesssion In"="COM11"}
  in  "# HVOF TC":i32=2
  in  "# HVOF Current Chan":i32=4
  out "TDMS error out":errorcluster
  out "TDMS file out":refnum<k34>
  in  "Sensor Indicator Tab Control":enum32{"Page 1", "Page 2", "Page 3", "Page 5"}(tab)
  out "T Sample":cluster{timestamp[], dbl[]}(graph)
  out "Delta T":cluster{timestamp[], dbl[]}(graph)
  out "T-W-out":dbl=17.150762268550952
  out "T-W-in":dbl=17.273451779340505
  out "Delta T":dbl=0.12268951078955226 format="%#_3g"
  out "T-Sample":dbl=16.92806090865619
  in  "Clear Data":bool
  out "O-P":dbl[unit](knob)=14.93 scale=0.0..450.0 scale format="%#_4g"
  out "Ar-P":dbl[unit](knob)=104.12 scale=0.0..450.0 scale format="%#_4g"
  out "Ar-m'  2":dbl[unit](knob)=-0.09 scale=0.0..450.0 scale format="%#_4g"
  out "O-F":dbl(knob)=-0.1 scale=0.0..450.0 scale format="%#_4g"
  out "Ar-T":dbl(slide)=18.33 scale=0.0..100.0
  out "O-T":dbl(slide)=18.45 scale=0.0..100.0
  out "Ar-m'":dbl[unit]=-0.1465155 format="%#_3f"
  out "O2-m'":dbl[unit]=-0.1302 format="%#_3f"
  out "O/F":dbl(knob)=87.17697597220514 scale=0.0..6.0
  out "F-m'":dbl[unit]=0.0018611133925148017 format="%#_3g"
  out "C-P":dbl(knob)=14.755946928632032 scale=0.0..60.0 scale format="%#_4g"
  out "PNP":dbl(knob)=-6.516446397140361 scale=0.0..60.0 scale format="%#_4g"
  out "W-m'":dbl[unit]=5637.227790905208 format="%#_3g"
  out "Heat loss to water":dbl[unit](knob)=2462845.9961641226
  out "Total Heat input":dbl[unit](knob)=119111.25712094731
  out "F-F":dbl(knob)=0.00021340766900836388 scale format="%#_4g"
  out "W-F":dbl(knob)=5.637227790905208 scale format="%#_4g"
  out "Ar-F":dbl[unit](knob)=-0.01 scale=0.0..450.0 scale format="%#_4g"
  out "O-m'":dbl[unit](knob)=-0.1 scale=0.0..450.0 scale format="%#_4g"
  out "SD- PNP?":dbl=0.5679065732287641 format="%#_3g"
  out "SD-C-P":dbl=0.7266970019796585 format="%#_3g"
  out "SD- F-F":dbl=0.0005978546529137135 format="%#_3g"
  out "SD- W-F":dbl=0.27493653666552775 format="%#_3g"
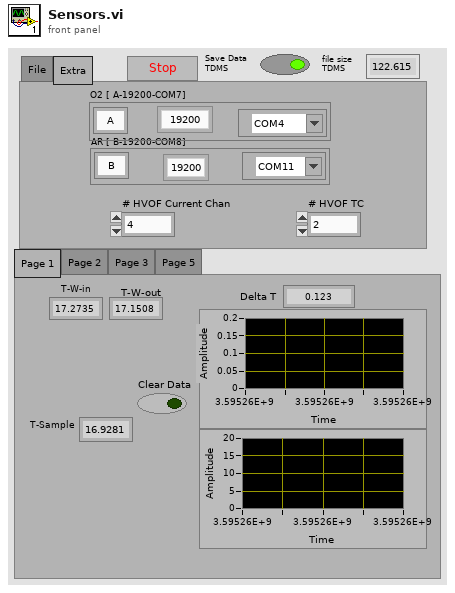
[diagram p1: front panel]
types:
  T1 = cluster{"Dynamic Data":dynamicdata, "Dynamic Data":dynamicdata, "Dynamic Data":dynamicdata, "Dynamic Data Type":dynamicdata}
  T2 = cluster{" ID":string, "Baud":enum8{"2400", "9600", "19200", "38400", "57600", "115200", "Unknown"}, "VISA Sesssion In":refnum<visa-resource-name>}
  T3 = cluster{" ID":string, "Baud ":enum8{"2400", "9600", "19200", "38400", "57600", "115200", "Unknown"}, "VISA Sesssion In":refnum<visa-resource-name>}
  T4 = enum16{"open", "open or create", "create or replace", "create", "open (read-only)"}
  T5 = cluster{"Absolute Pressure":bool, "Gauge/Diff. Pressure":bool, "Barometric Pressure":bool, "Temperature":bool, "Volumetric":bool, "Mass":bool, "Setpoint":bool, "Valve Drive":bool, "Totalizer":bool, "Totalizer Timer":bool, "Totalizer Average Flow":bool, "Totalizer Peak Flow":bool, "Gas Selected":bool, "Tot. Timer Format":u16}
  T6 = cluster{"Abs. Pressure":string, "Gauge/Diff. Press.":string, "Barometric Press.":string, "Temperature":string, "Volume":string, "Mass":string, "Setpoint":string, "Valve Drive":string, "Totalizer":string, "Tot. Timer":string, "Tot. Avg. Flow":string, "Tot. Peak Flow":string}
  T7 = cluster{"Absolute Pressure":dbl, "Gauge/Diff. Pressure":dbl, "Barometric Pressure":dbl, "Temperature":dbl, "Volumetric Flow":dbl, "Mass Flow":dbl, "Setpoint":dbl, "Valve Drive":dbl, "Totalizer":dbl, "[hr]":dbl, "[min]":dbl, "[sec]":dbl, "Totalizer Average Flow":dbl, "Totalizer Peak Flow":dbl, "Gas selected":string}
  T8 = cluster{dynamicdata, dynamicdata, "Arithmetic Mean":dynamicdata, "Dynamic Data Type":dynamicdata}
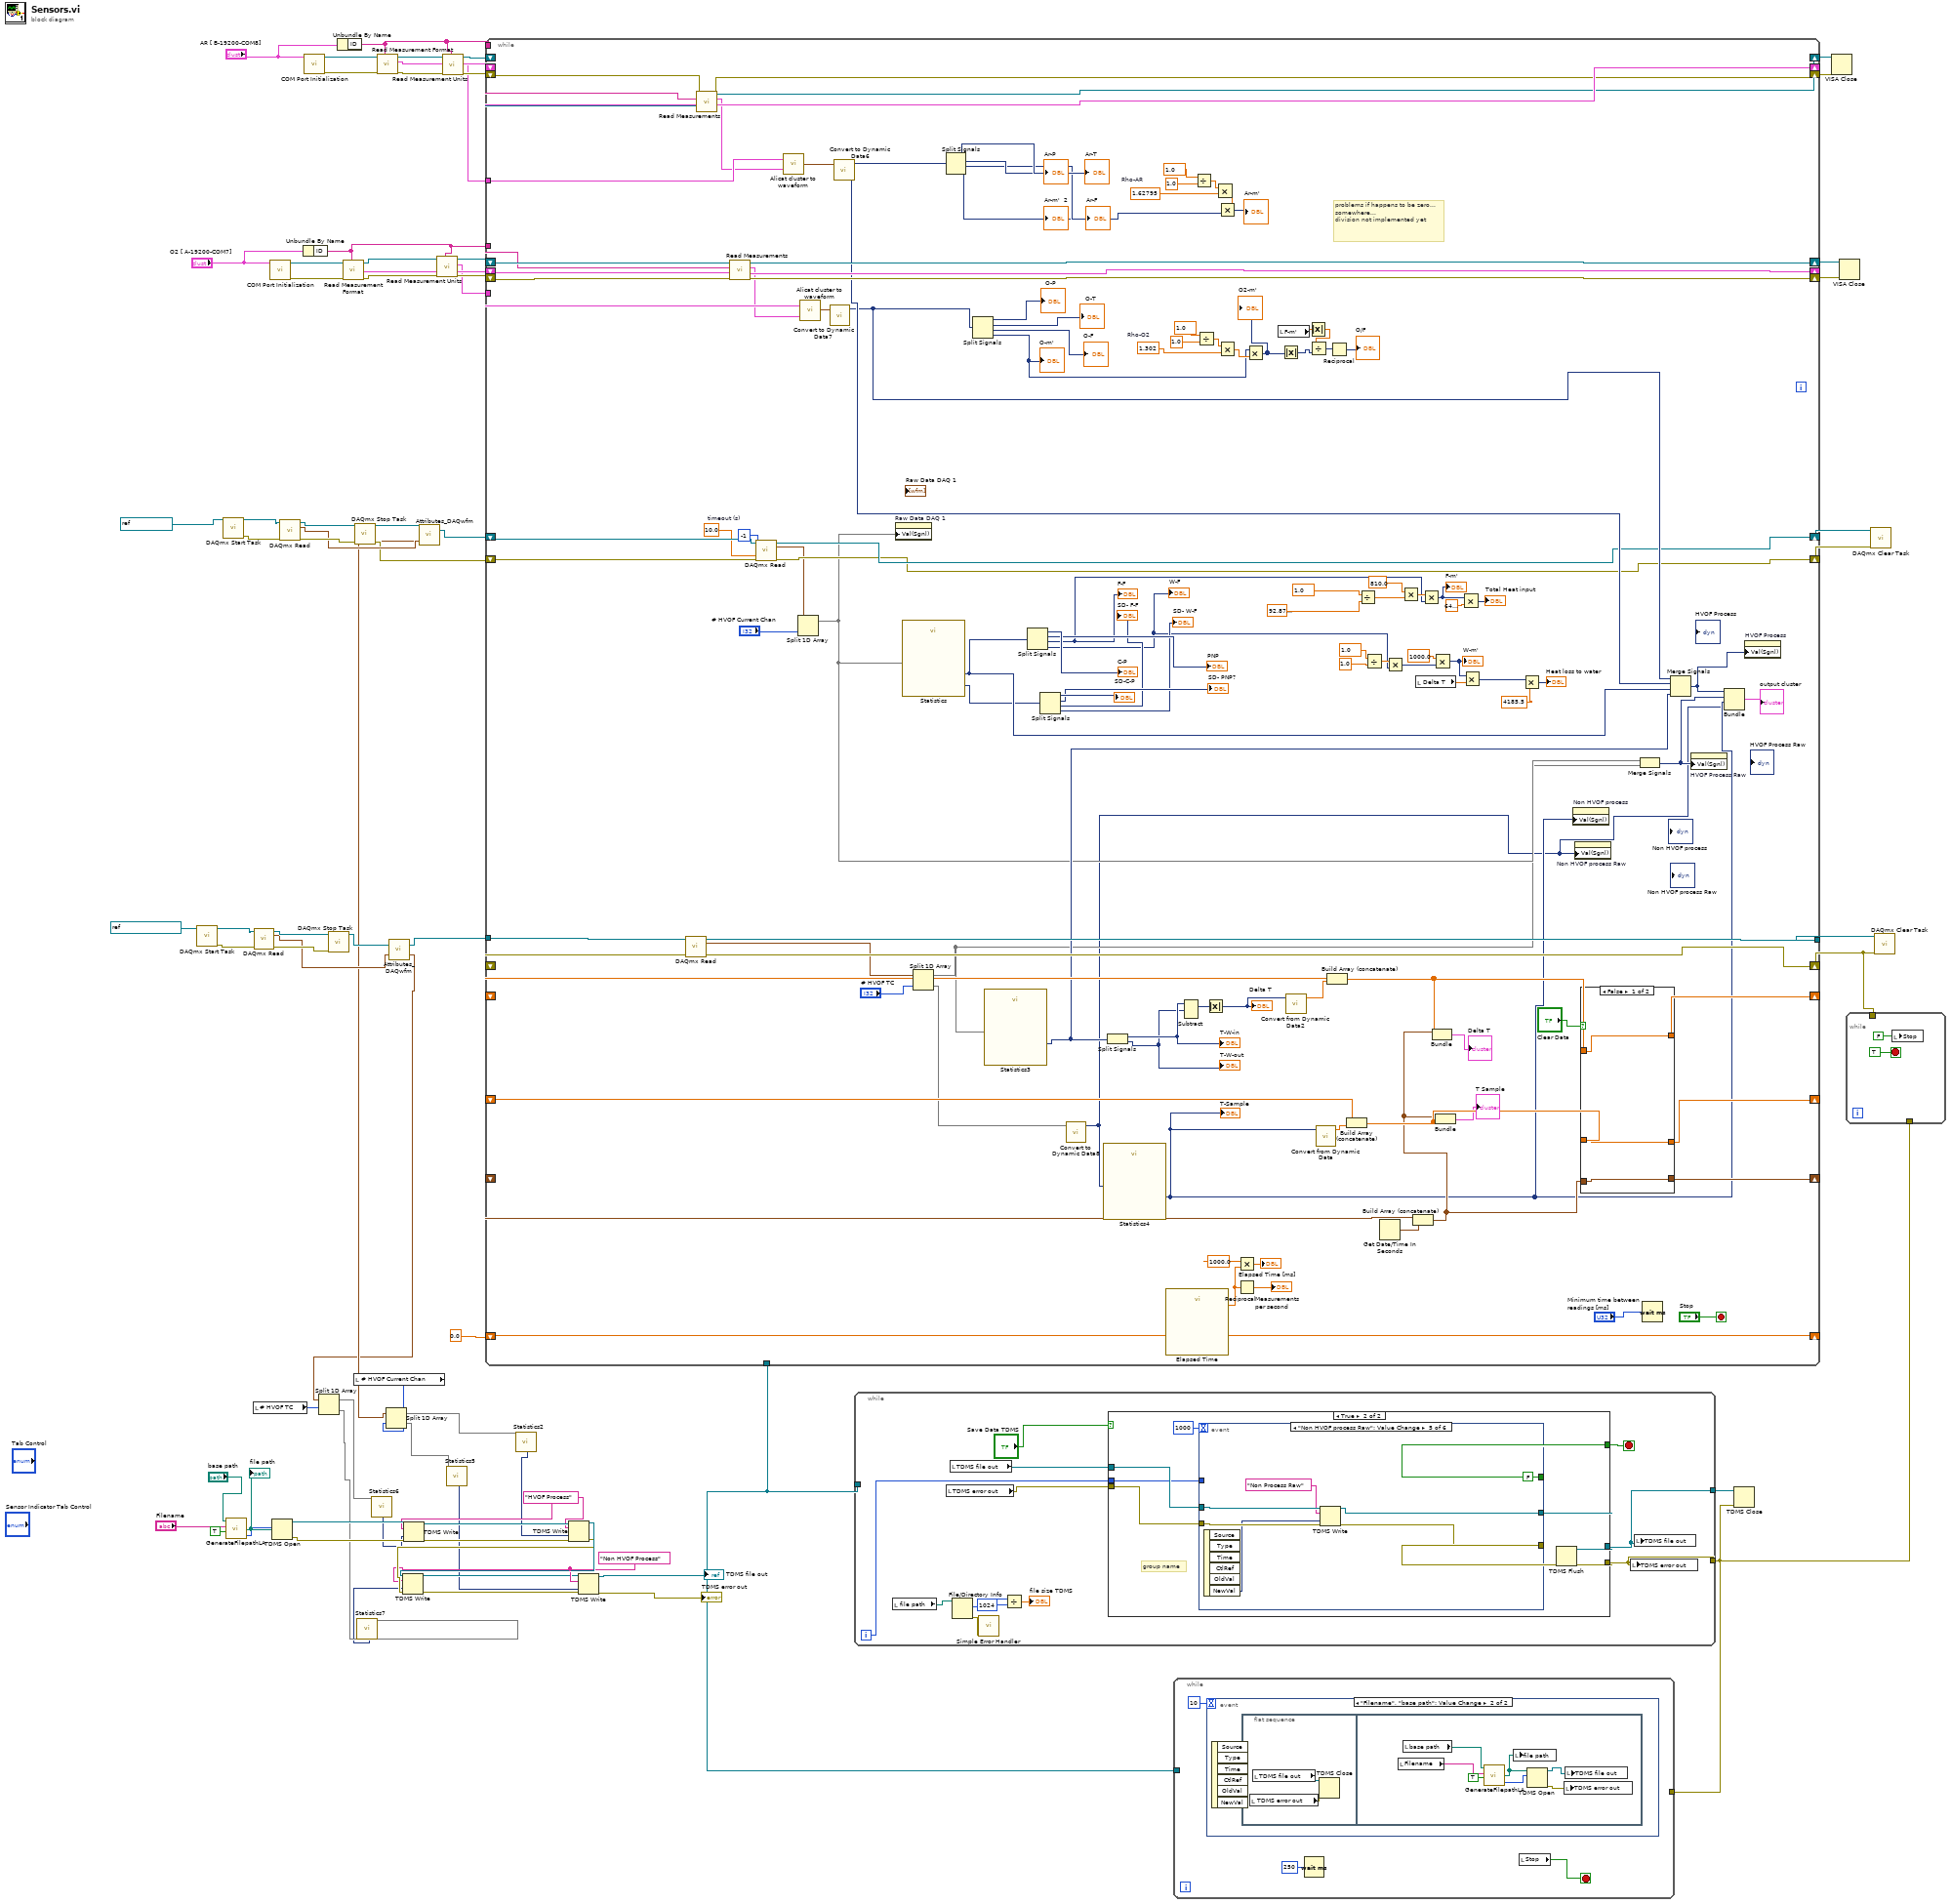
[diagram p0: block diagram]
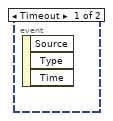
[diagram p2: hidden frame]
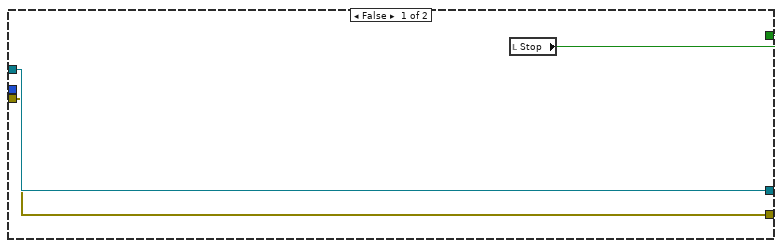
[diagram p3: hidden frame]
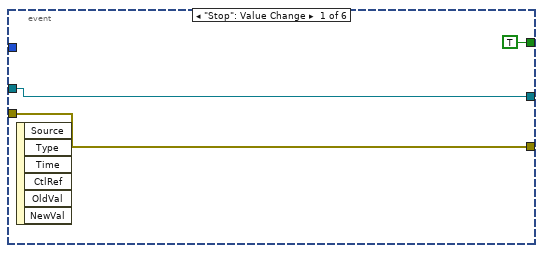
[diagram p4: hidden frame]
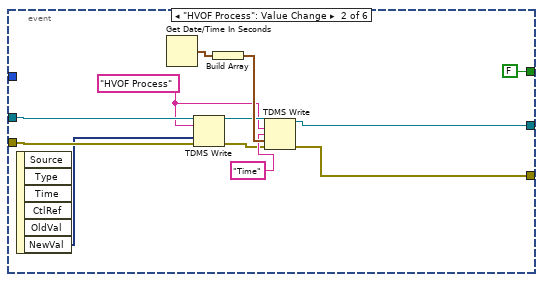
[diagram p5: hidden frame]
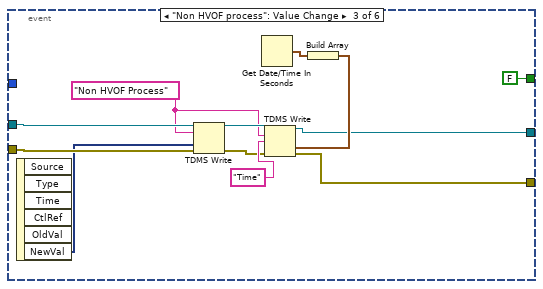
[diagram p6: hidden frame]
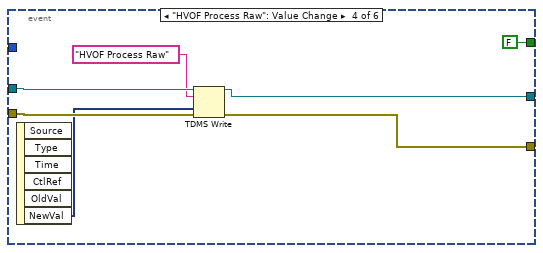
[diagram p7: hidden frame]
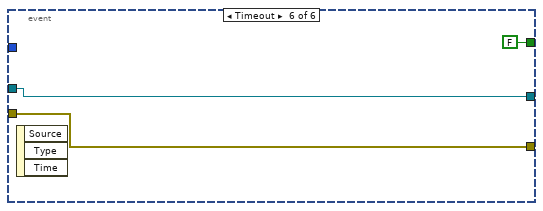
[diagram p8: hidden frame]
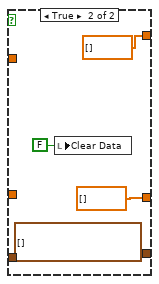
[diagram p9: hidden frame]
diagram:
  w12 = "Non HVOF Process" ("group name in (Untitled)")
  w20 = "HVOF Process" ("group name in (Untitled)")
  n1 = call <vilib>:"DAQmx Start Task.vi"("task/channels in"=refnum<k21> "Temperature_1" ("task out")) -> ("task out"=w27:refnum<k21>, "error out"=w28:errorcluster)  [unwired: 13 in]
  n2 = call <vilib>:"DAQmx Start Task.vi"("task/channels in"=refnum<k21> "Current_1") -> ("task out"=w40:refnum<k21>, "error out"=w39:errorcluster)  [unwired: 13 in]
  n3 = call "GenerateFilepathLA.vi"("Auto Date folder"=TRUE, "Filename"="Filename", "base path"="base path") -> ("operation (0:open)"=w60:T4, "file path"=w61:path)  [unwired: 1 in, 1 out]
  "file path" <- w61
  n4 = local read "# HVOF TC"() -> (w19:i32)
  n5 = call-poly <vilib>:"DAQmx Read.vi"("task/channels in"=w27, "error in"=w28) -> ("task out"=w29:refnum<k21>, "data"=w21:waveform(dbl)[], "error out"=w30:errorcluster)  [unwired: 11 in]
  n6 = call "COM Port Initialization.vi"("Communication Settings"="O2 [ A-19200-COM7]") -> ("error out"=w76:errorcluster, "VISA Session Out"=w77:refnum<visa-resource-name>)  [unwired: 9 in]
  n7 = TDMS Open(10:w60, 11:w61) -> (0:w31:errorcluster, 3:w32:refnum<k34>)  [unwired: 5 in]
  n8 = call-poly <vilib>:"DAQmx Read.vi"("task/channels in"=w40, "error in"=w39) -> ("task out"=w38:refnum<k21>, "data"=w35:waveform(dbl)[], "error out"=w37:errorcluster)  [unwired: 11 in]
  n9 = Unbundle By Name("O2 [ A-19200-COM7]") -> ("ID"=w44:string)
  n10 = call "COM Port Initialization.vi"("Communication Settings"="AR [ B-19200-COM8]") -> ("error out"=w75:errorcluster, "VISA Session Out"=w74:refnum<visa-resource-name>)  [unwired: 9 in]
  n11 = call <vilib>:"DAQmx Stop Task.vi"("task/channels in"=w29, "error in"=w30) -> ("task out"=w23:refnum<k21>)  [unwired: 12 in, 1 out]
  n12 = Unbundle By Name("AR [ B-19200-COM8]") -> ("ID"=w49:string)
  n13 = call "Read Measurement Format.vi"("Unit ID (A)"=w44, "error in"=w76, "VISA Session In"=w77) -> ("error out"=w46:errorcluster, "Data Frame Format"=w71:T5, "VISA Session Out"=w48:refnum<visa-resource-name>)  [unwired: 6 in]
  n14 = local read "# HVOF Current Chan"() -> (w18:i32)
  n15 = call <vilib>:"DAQmx Stop Task.vi"("task/channels in"=w38, "error in"=w37) -> ("task out"=w36:refnum<k21>, "error out"=w34:errorcluster)  [unwired: 12 in]
  n16 = call "Read Measurement Format.vi"("Unit ID (A)"=w49, "error in"=w75, "VISA Session In"=w74) -> ("error out"=w52:errorcluster, "Data Frame Format"=w70:T5, "VISA Session Out"=w53:refnum<visa-resource-name>)  [unwired: 6 in]
  n17 = call "Attributes_DAQwfm.vi"("data"=w21, "Refnum in"=w23) -> ("Array"=w16:waveform(dbl)[], "Refnum in 2"=w22:refnum<k21>)
  n18 = Split 1D Array(array=w16, index=w19) -> (first subarray=w1:waveform(dbl)[], second subarray=w4:waveform(dbl)[])
  n19 = call "Statistics7"("Signals"=w4) -> ("Arithmetic Mean"=w3:dynamicdata)  [unwired: 24 in, 2 out]
  n20 = call "Statistics6"("Signals"=w1) -> ("Arithmetic Mean"=w5:dynamicdata)  [unwired: 24 in, 2 out]
  n21 = TDMS Write(0:w32, 5:w20, 9:w5, 11:w31) -> (4:w25:refnum<k34>, 15:w24:errorcluster)  [unwired: 2 in, 2 out]
  n22 = call "Attributes_DAQwfm.vi"("data"=w35, "Refnum in"=w36) -> ("Array"=w17:waveform(dbl)[], "Refnum in 2"=w33:refnum<k21>)
  n23 = Split 1D Array(array=w17, index=w18) -> (first subarray=w8:waveform(dbl)[], second subarray=w6:waveform(dbl)[])
  n24 = call "Read Measurement Units.vi"("Unit ID (A)"=w44, "error in"=w46, "VISA Session In"=w48) -> ("error out"=w45:errorcluster, "Measurement Units"=w42:T6, "VISA Session Out"=w47:refnum<visa-resource-name>)  [unwired: 5 in, 1 out]
  n25 = call "Read Measurement Units.vi"("Unit ID (A)"=w49, "error in"=w52, "VISA Session In"=w53) -> ("error out"=w50:errorcluster, "Measurement Units"=w43:T6, "VISA Session Out"=w51:refnum<visa-resource-name>)  [unwired: 5 in, 1 out]
  n26 = call "Statistics5"("Signals"=w6) -> ("Arithmetic Mean"=w2:dynamicdata)  [unwired: 24 in, 2 out]
  n27 = call "Statistics2"("Signals"=w8) -> ("Arithmetic Mean"=w7:dynamicdata)  [unwired: 24 in, 2 out]
  n28 = TDMS Write(0:w25, 5:w20, 9:w7, 11:w24) -> (4:w15:refnum<k34>, 15:w14:errorcluster)  [unwired: 2 in, 2 out]
  n29 = TDMS Write(0:w15, 5:w12, 9:w3, 11:w14) -> (4:w10:refnum<k34>, 15:w9:errorcluster)  [unwired: 2 in, 2 out]
  n30 = TDMS Write(0:w10, 5:w12, 9:w2, 11:w9) -> (4:w11:refnum<k34>, 15:→"TDMS error out":errorcluster)  [unwired: 2 in, 2 out]
  "TDMS file out" <- w11
  n31 = while {
    shift-right: [w197] -> w69
    shift-left: w47 -> [w201]
    shift-right: [w192] -> _
    shift-left: w71 -> [w200]
    shift-right: [w191] -> w68
    shift-left: w51 -> [w196]
    tunnel: w44 -> [w199]
    tunnel: w49 -> [w194]
    shift-right: [w193] -> _
    shift-left: w70 -> [w195]
    shift-right: [w187] -> w66
    shift-left: w50 -> [w190]
    shift-right: [w188] -> w67
    shift-left: w45 -> [w189]
    shift-right: [w182] -> _
    shift-left: 0.0 ("Set Start Time (s)") -> [w183]
    shift-right: [w168] -> _
    shift-left: _ -> [w180]
    shift-right: [w177] -> w58
    shift-left: w33 -> [w174]
    shift-right: [w176] -> w57
    shift-left: w34 -> [w175]
    shift-right: [w169] -> _
    shift-left: _ -> [w172]
    shift-right: [w162] -> _
    shift-left: _ -> [w163]
    tunnel: [w165] -> w55
    shift-right: [w160] -> w54
    shift-left: _ -> [w166]
    tunnel: w22 -> [w159]
    tunnel: w43 -> [w158]
    tunnel: w42 -> [w157]
    tunnel: w11 -> [_]
    stop <- "Stop" stop-if-true
    w105 = dbl[unit] 1.62795  # Rho-AR
    w120 = dbl[unit] 1.302  # Rho-O2
    w156 = 10.0  # timeout (s)
    # "problems if happens to be zero...somewhere...\ndivision not implemented yet"
    n32 = call-poly <vilib>:"DAQmx Read.vi"("task/channels in"=w159, "error in"=w166) -> ("task out"=w165:refnum<k21>, "data"=w89:waveform(dbl)[], "error out"=w160:errorcluster)  [unwired: 11 in]
    n33 = call "Read Measurements.vi"("error in"=w190, "Data Frame Format In"=w195, "Unit ID (A)"=w194, "VISA Session In"=w196) -> ("error out"=w187:errorcluster, "Data Frame Format Out"=w193:T5, "Data Cluster"=w110:T7, "VISA Session Out"=w191:refnum<visa-resource-name>)  [unwired: 4 out]
    n34 = call "Read Measurements.vi"("error in"=w189, "Data Frame Format In"=w200, "Unit ID (A)"=w199, "VISA Session In"=w201) -> ("error out"=w188:errorcluster, "Data Frame Format Out"=w192:T5, "Data Cluster"=w98:T7, "VISA Session Out"=w197:refnum<visa-resource-name>)  [unwired: 4 out]
    n35 = call-poly <vilib>:"DAQmx Read.vi"("task/channels in"=w174, "number of samples per channel"=-1, "timeout"=w156, "error in"=w175) -> ("task out"=w177:refnum<k21>, "data"=w127:waveform(dbl)[], "error out"=w176:errorcluster)  [unwired: 9 in]
    n36 = call "Alicat cluster to waveform.vi"("Data Cluster in"=w110, "Measurement Units in"=w158) -> ("Array"=w99:waveform(dbl)[])
    n37 = Split 1D Array(array=w127, index="# HVOF Current Chan") -> (first subarray=w82:waveform(dbl)[])  [unwired: 1 out]
    n38 = call "Alicat cluster to waveform.vi"("Data Cluster in"=w98, "Measurement Units in"=w157) -> ("Array"=w97:waveform(dbl)[])
    n39 = call "Convert to Dynamic Data7"("Array of Waveforms"=w97) -> ("Dynamic Data Type"=w178:dynamicdata)  [unwired: 3 in]
    n40 = call "Convert to Dynamic Data6"("Array of Waveforms"=w99) -> ("Dynamic Data Type"=w179:dynamicdata)  [unwired: 3 in]
    n41 = property on="Raw Data DAQ 1" class="WFGraph (strict)"("Val(Sgnl)"=w82) -> ()  [unwired: 2 in, 2 out]
    n42 = call "Statistics"("Signals"=w82) -> ("Standard Dev"=w154:dynamicdata, "Arithmetic Mean"=w173:dynamicdata)  [unwired: 24 in, 1 out]
    n43 = Split 1D Array(array=w89, index="# HVOF TC") -> (first subarray=w81:waveform(dbl)[], second subarray=w86:waveform(dbl)[])
    n44 = Split Signals(w179) -> (→"Ar-P":dynamicdata, →"Ar-T":dynamicdata, →"Ar-F":dynamicdata, w101:dynamicdata)  [unwired: 4 in]
    "Ar-m'  2" <- w101
    n45 = Split Signals(w178) -> (→"O-P":dynamicdata, →"O-T":dynamicdata, →"O-F":dynamicdata, w118:dynamicdata)  [unwired: 4 in]
    "O-m'" <- w118
    n46 = call "Statistics3"("Signals"=w81) -> ("Arithmetic Mean"=w83:dynamicdata)  [unwired: 24 in, 2 out]
    n47 = Split Signals(w173) -> (→"C-P":dynamicdata, →"PNP":dynamicdata, w129:dynamicdata, w128:dynamicdata)  [unwired: 4 in]
    "W-F" <- w128
    "F-F" <- w129
    n48 = Split Signals(w154) -> (→"SD-C-P":dynamicdata, →"SD- PNP?":dynamicdata, →"SD- F-F":dynamicdata, →"SD- W-F":dynamicdata)  [unwired: 4 in]
    n49 = call "Convert to Dynamic Data8"("Array of Waveforms"=w86) -> ("Dynamic Data Type"=w79:dynamicdata)  [unwired: 3 in]
    n50 = call "Statistics4"("Signals"=w79) -> ("Arithmetic Mean"=w84:dynamicdata)  [unwired: 24 in, 2 out]
    "T-Sample" <- w84
    n51 = Split Signals(w83) -> (w95:dynamicdata, w87:dynamicdata)  [unwired: 2 in]
    "T-W-out" <- w87
    "T-W-in" <- w95
    n52 = call "Elapsed Time"("Set Start Time (s)"=w183) -> ("Get Start Time (s)"=w182:dbl, "Elapsed Time (s)"=w186:dbl)  [unwired: 11 in, 6 out]
    n53 = Subtract(1:w87, 2:w95) -> (0:w96:dynamicdata)  [unwired: 1 in, 1 out]
    n54 = Divide(x=dbl[unit] 1.0, y=dbl[unit] 1.0) -> (x/y=w103:dbl)
    n55 = Divide(x=dbl[unit] 1.0, y=dbl[unit] 1.0) -> (x/y=w121:dbl)
    n56 = Absolute Value(x=w96) -> (abs(x)=w94:dynamicdata)
    "Delta T" <- w94
    n57 = Multiply(x=w103, y=w105) -> (x*y=w102:dbl[unit])
    n58 = Multiply(x=w102, y=w101) -> (x*y=→"Ar-m'":dynamicdata)
    n59 = Multiply(x=w121, y=w120) -> (x*y=w119:dbl[unit])
    n60 = Multiply(x=1000.0, y=w186) -> (x*y=→"Elapsed Time [ms]":dbl)
    n61 = Reciprocal(x=w186) -> (1/x=→"Measurements\nper second":dbl)
    n62 = Multiply(x=w118, y=w119) -> (x*y=w113:dynamicdata)
    "O2-m'" <- w113
    n63 = local read "F-m'"() -> (w115:dbl[unit])
    n64 = Absolute Value(x=w113) -> (abs(x)=w112:dynamicdata)
    n65 = call "Convert from Dynamic Data2"("Dynamic Data Type"=w94) -> ("Scalar"=w93:dbl)  [unwired: 3 in]
    n66 = Absolute Value(x=w115) -> (abs(x)=w114:dbl[unit])
    n67 = Divide(x=w114, y=w112) -> (x/y=w117:dynamicdata)
    n68 = call "Convert from Dynamic Data"("Dynamic Data Type"=w84) -> ("Scalar"=w92:dbl)  [unwired: 3 in]
    n69 = Build Array (concatenate)(w180, w93) -> (w171:dbl[])
    n70 = Reciprocal(x=w117) -> (1/x=→"O/F":dynamicdata)
    n71 = Build Array (concatenate)(w172, w92) -> (w170:dbl[])
    n72 = Divide(x=dbl[unit] 1.0, y=dbl[unit] 92.87999999999998) -> (x/y=w135:dbl[unit])
    n73 = Divide(x=dbl[unit] 1.0, y=dbl[unit] 1.0) -> (x/y=w145:dbl)
    n74 = Get Date/Time In Seconds() -> (seconds since 1Jan1904=w164:timestamp)
    n75 = Multiply(x=w145, y=w128) -> (x*y=w130:dynamicdata)
    n76 = Multiply(x=dbl[unit] 810.0 ("Rhol-F"), y=w135) -> (x*y=w137:dbl[unit])
    n77 = Build Array (concatenate)(w163, w164) -> (w161:timestamp[])
    n78 = local read "Delta T"() -> (w132:dbl)
    n79 = Multiply(x=w137, y=w129) -> (x*y=w134:dynamicdata)
    "F-m'" <- w134
    n80 = Bundle(w161, w171) -> (→"Delta T":cluster{timestamp[], dbl[]})  [unwired: 1 in]
    n81 = Multiply(x=dbl[unit] 1000.0 ("y"), y=w130) -> (x*y=w142:dynamicdata)
    "W-m'" <- w142
    n82 = Bundle(w161, w170) -> (→"T Sample":cluster{timestamp[], dbl[]})  [unwired: 1 in]
    n83 = Multiply(x=w134, y=dbl[unit] 64000000.0) -> (x*y=→"Total Heat input":dynamicdata)
    n84 = Multiply(x=w142, y=w132) -> (x*y=w143:dynamicdata)
    n85 = Multiply(x=w143, y=dbl[unit] 4185.5) -> (x*y=→"Heat loss to water":dynamicdata)
    n86 = property on="Non HVOF process" class="WFGraph (strict)"("Val(Sgnl)"=w84) -> ()  [unwired: 2 in, 2 out]
    n87 = property on="Non HVOF process Raw" class="WFGraph (strict)"("Val(Sgnl)"=w79) -> ()  [unwired: 2 in, 2 out]
    n88 = case shown="False" "Clear Data" {
      tunnel: w171 -> [w204 _]
      tunnel: w170 -> [w205 _]
      tunnel: [w205 dbl[] []] -> w169
      tunnel: [w204 dbl[] []] -> w168
      tunnel: [w203 timestamp[] []] -> w162
      tunnel: w161 -> [w203 _]
      frame False {
      }
      frame True {
        n89 = local write "Clear Data"(FALSE ("Clear Data")) -> ()
      }
    }
    n90 = Merge Signals(w82, w81) -> (w80:dynamicdata)
    n91 = Wait (ms)(milliseconds to wait="Minimum time between \nreadings [ms]") -> ()  [unwired: 1 out]
    n92 = Merge Signals(w178, w179, w173, w83) -> (w85:dynamicdata)
    n93 = property on="HVOF Process Raw" class="WFGraph (strict)"("Val(Sgnl)"=w80) -> ()  [unwired: 2 in, 2 out]
    n94 = Bundle(w85, w80, "Arithmetic Mean"=w84, "Dynamic Data Type"=w79) -> (→"output cluster":T8)  [unwired: 1 in]
    n95 = property on="HVOF Process" class="WFGraph (strict)"("Val(Sgnl)"=w85) -> ()  [unwired: 2 in, 2 out]
  }
  n96 = while {
    tunnel: w11 -> [_]
    tunnel: [w218] -> w59
    tunnel: [w217] -> w56
    i -> [w211]
    stop <- w210 stop-if-true
    n97 = local read "file path"() -> (w215:path)
    n98 = local read "TDMS error out"() -> (w219:errorcluster)
    n99 = local read "TDMS file out"() -> (w220:refnum<k34>)
    n100 = File/Directory Info(path=w215) -> (size=w213:i64, error out=w216:errorcluster)  [unwired: 1 in, 5 out]
    n101 = call <vilib>:"Simple Error Handler.vi"("error in (no error)"=w216) -> ()  [unwired: 1 in, 8 out]
    n102 = Divide(x=w213, y=i64 1024) -> (x/y=→"file size TDMS":dbl)
    n103 = case shown="True" "Save Data TDMS" {
      tunnel: w220 -> [w224 w231]
      tunnel: w219 -> [w223 w230]
      tunnel: [w224 w233] -> w218
      tunnel: [w223 w232] -> w217
      tunnel: w211 -> [_ w229]
      tunnel: [w222 w226] -> w210
      frame False {
        n104 = local read "Stop"() -> (w222:bool)
      }
      frame True {
        # "group name"
        n105 = event shown="[4] \"Non HVOF process Raw\": Value Change" {
          selector: _ -> [_ _ _ _ _ _]
          dyn-events: _ -> [_ _ _ _ _ _]
          timeout: 1000 -> [_ _ _ _ _ _]
          tunnel: w231 -> [w236 w248 w260 w267 w274 w277]
          tunnel: w230 -> [w235 w247 w259 w266 w273 w276]
          tunnel: [w236 w240 w252 w264 w271 w277] -> w228
          tunnel: [w235 w239 w251 w263 w270 w276] -> w227
          tunnel: w229 -> [_ _ _ _ _ _]
          tunnel: [TRUE FALSE FALSE FALSE FALSE FALSE] -> w226
          event "Stop": Value Change {
            n106 = event-data() -> ()  [unwired: 1 in, 6 out]
          }
          event "HVOF Process": Value Change {
            w237 = "HVOF Process" ("group name in (Untitled)")
            n107 = event-data() -> ("NewVal"=w246:dynamicdata)  [unwired: 1 in, 5 out]
            n108 = Get Date/Time In Seconds() -> (seconds since 1Jan1904=w245:timestamp)
            n109 = TDMS Write(0:w248, 5:w237, 9:w246, 11:w247) -> (4:w242:refnum<k34>, 15:w241:errorcluster)  [unwired: 2 in, 2 out]
            n110 = Build Array(w245) -> (w244:timestamp[])
            n111 = TDMS Write(0:w242, 5:w237, 7:"Time" ("property names"), 9:w244, 11:w241) -> (4:w240:refnum<k34>, 15:w239:errorcluster)  [unwired: 1 in, 2 out]
          }
          event "Non HVOF process": Value Change {
            w249 = "Non HVOF Process" ("group name in (Untitled)")
            n112 = event-data() -> ("NewVal"=w258:dynamicdata)  [unwired: 1 in, 5 out]
            n113 = TDMS Write(0:w260, 5:w249, 9:w258, 11:w259) -> (4:w254:refnum<k34>, 15:w253:errorcluster)  [unwired: 2 in, 2 out]
            n114 = Get Date/Time In Seconds() -> (seconds since 1Jan1904=w257:timestamp)
            n115 = Build Array(w257) -> (w256:timestamp[])
            n116 = TDMS Write(0:w254, 5:w249, 7:"Time" ("property names"), 9:w256, 11:w253) -> (4:w252:refnum<k34>, 15:w251:errorcluster)  [unwired: 1 in, 2 out]
          }
          event "HVOF Process Raw": Value Change {
            n117 = event-data() -> ("NewVal"=w265:dynamicdata)  [unwired: 1 in, 5 out]
            n118 = TDMS Write(0:w267, 5:"HVOF Process Raw" ("group name in (Untitled)"), 9:w265, 11:w266) -> (4:w264:refnum<k34>, 15:w263:errorcluster)  [unwired: 2 in, 2 out]
          }
          event "Non HVOF process Raw": Value Change {
            n119 = event-data() -> ("NewVal"=w272:dynamicdata)  [unwired: 1 in, 5 out]
            n120 = TDMS Write(0:w274, 5:"Non Process Raw" ("group name in (Untitled)"), 9:w272, 11:w273) -> (4:w271:refnum<k34>, 15:w270:errorcluster)  [unwired: 2 in, 2 out]
          }
          event Timeout {
            n121 = event-data() -> ()  [unwired: 1 in, 3 out]
          }
        }
        n122 = TDMS Flush(4:w227, 7:w228) -> (0:w232:errorcluster, 3:w233:refnum<k34>)
      }
    }
    n123 = local write "TDMS error out"(w217) -> ()
    n124 = local write "TDMS file out"(w218) -> ()
  }
  n125 = while {
    tunnel: w11 -> [_]
    tunnel: w56 -> [_]
    stop <- w280 stop-if-true
    n126 = event shown="[1] \"Filename\", \"base path\": Value Change" {
      selector: _ -> [_ _]
      dyn-events: _ -> [_ _]
      timeout: 10 -> [_ _]
      event Timeout {
        n127 = event-data() -> ()  [unwired: 1 in, 3 out]
      }
      event "Filename", "base path": Value Change {
        n128 = event-data() -> ()  [unwired: 1 in, 6 out]
        n129 = flat-sequence {
          frame #0 {
            n130 = local read "TDMS error out"() -> (w282:errorcluster)
            n131 = local read "TDMS file out"() -> (w281:refnum<k34>)
            n132 = TDMS Close(8:w282, 11:w281) -> ()  [unwired: 2 out]
          }
          frame #1 {
            n133 = local read "Filename"() -> (w289:string)
            n134 = local read "base path"() -> (w288:path)
            n135 = call "GenerateFilepathLA.vi"("Auto Date folder"=TRUE, "Filename"=w289, "base path"=w288) -> ("operation (0:open)"=w285:T4, "file path"=w287:path)  [unwired: 1 in, 1 out]
            n136 = local write "file path"(w287) -> ()
            n137 = TDMS Open(10:w285, 11:w287) -> (0:w283:errorcluster, 3:w284:refnum<k34>)  [unwired: 5 in]
            n138 = local write "TDMS error out"(w283) -> ()
            n139 = local write "TDMS file out"(w284) -> ()
          }
        }
      }
    }
    n140 = Wait (ms)(milliseconds to wait=u32 250) -> ()  [unwired: 1 out]
    n141 = local read "Stop"() -> (w280:bool)
  }
  n142 = TDMS Close(8:w56, 11:w59) -> ()  [unwired: 2 out]
  n143 = VISA Close(VISA resource name=w68, error in (no error)=w66) -> ()  [unwired: 1 out]
  n144 = VISA Close(VISA resource name=w69, error in (no error)=w67) -> ()  [unwired: 1 out]
  n145 = while {
    tunnel: w56 -> [_]
    tunnel: w54 -> [_]
    stop <- TRUE stop-if-true
    n146 = local write "Stop"(FALSE ("stop_vi")) -> ()
  }
  n147 = call <vilib>:"DAQmx Clear Task.vi"("task in"=w58, "error in"=w57) -> ()  [unwired: 13 in, 1 out]
  n148 = call <vilib>:"DAQmx Clear Task.vi"("task in"=w55, "error in"=w54) -> ()  [unwired: 13 in, 1 out]
